vi "Pick and Place Pick Up Tool.vi"   [LabVIEW 2016]
uses:
  Drivers/Aerotech A3200/Aerotech VIs.lvlib
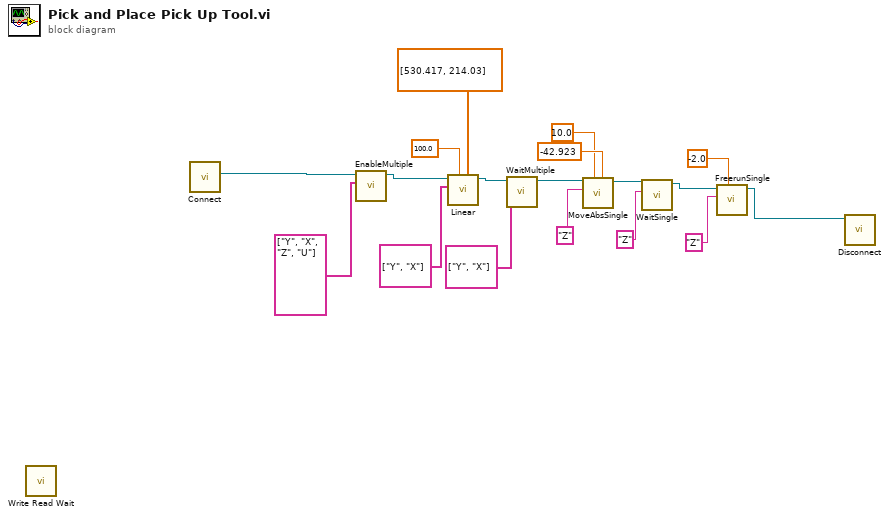
[diagram p0: block diagram]
diagram:
  n1 = call "Write Read Wait.vi"() -> ()  [unwired: 15 in, 1 out]
  n2 = call "Connect.vi"() -> ("controller"=w18:refnum<k24>)  [unwired: 10 in, 1 out]
  n3 = call "EnableMultiple.vi"("axis names"=string[] ["Y", "X", "Z", "U"], "controller in"=w18) -> ("controller out"=w16:refnum<k24>)  [unwired: 8 in, 1 out]
  n4 = call "Linear.vi"("distances"=dbl[] [530.417, 214.03], "speed"=100.0, "axis names"=string[] ["Y", "X"], "controller in"=w16) -> ("controller out"=w11:refnum<k24>)  [unwired: 6 in, 1 out]
  n5 = call "WaitMultiple.vi"("axis names"=string[] ["Y", "X"], "controller in"=w11) -> ("controller out"=w10:refnum<k24>)  [unwired: 7 in, 2 out]
  n6 = call "MoveAbsSingle.vi"("position"=-42.923, "speed"=10.0, "axis name"="Z", "controller in"=w10) -> ("controller out"=w6:refnum<k24>)  [unwired: 6 in, 1 out]
  n7 = call "WaitSingle.vi"("axis name"="Z", "controller in"=w6) -> ("controller out"=w4:refnum<k24>)  [unwired: 7 in, 2 out]
  n8 = call "FreerunSingle.vi"("speed"=-2.0, "axis name"="Z", "controller in"=w4) -> ("controller out"=w1:refnum<k24>)  [unwired: 7 in, 1 out]
  n9 = call "Disconnect.vi"("controller"=w1) -> ()  [unwired: 10 in, 1 out]
